vi "Pre Launch Init.vi"(11 "Nested in":refnum<class "Measurement GEN.lvclass">) -> (0 "error out":errorcluster, 3 "Nested out":refnum<class "Measurement GEN.lvclass">)   [LabVIEW 2020, in "Measurement GEN.lvlib" / "Measurement GEN.lvclass"]
doc: "(<B>Filename</B>: Actor Framework.lvlib:Actor.lvclass:Pre Launch Init.vi)\n\nDefines behavior that occurs after the Launch Nested Actor method is invoked but before the actor's Actor Core method begins running.\n\nBy default, this method does nothing. A descendant class may override it to define behavior."
uses:
  Measurement GEN.lvclass
  Measurement GEN.lvclass/Measurement GEN.ctl
  <vilib>/ActorFramework/Actor/Actor.lvclass
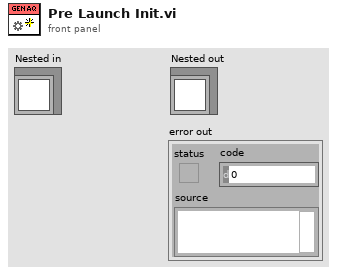
[diagram p1: front panel]
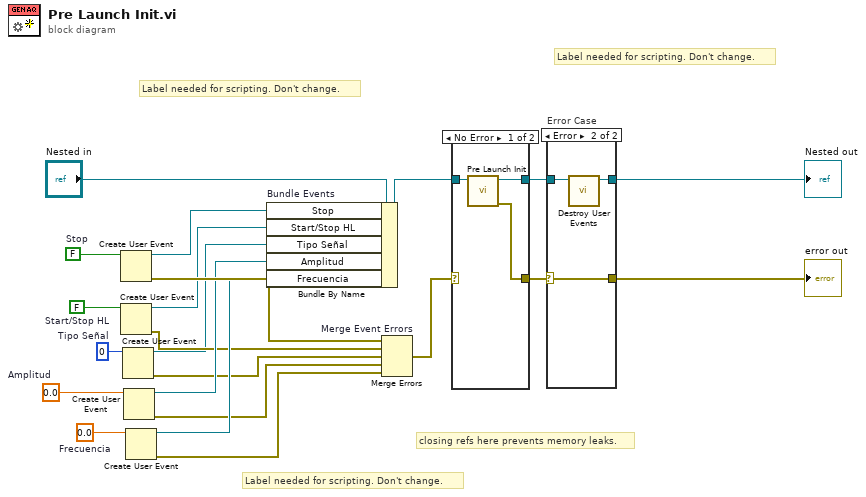
[diagram p0: block diagram]
diagram:
  w2 = u16 0  # Tipo Señal
  w11 = 0.0  # Frecuencia
  w12 = 0.0  # Amplitud
  w13 = FALSE  # Start/Stop HL
  w21 = FALSE  # Stop
  # "Label needed for scripting. Don't change."
  # "Label needed for scripting. Don't change."
  # "Label needed for scripting. Don't change."
  # "closing refs here prevents memory leaks."
  n1 = Create User Event(user event datatype=w21) -> (user event=w10:refnum<user-event>, error out=w20:errorcluster)  [unwired: 1 in]
  n2 = Create User Event(user event datatype=w13) -> (user event=w9:refnum<user-event>, error out=w6:errorcluster)  [unwired: 1 in]
  n3 = Create User Event(user event datatype=w2) -> (user event=w1:refnum<user-event>, error out=w5:errorcluster)  [unwired: 1 in]
  n4 = Create User Event(user event datatype=w12) -> (user event=w8:refnum<user-event>, error out=w4:errorcluster)  [unwired: 1 in]
  n5 = Create User Event(user event datatype=w11) -> (user event=w7:refnum<user-event>, error out=w3:errorcluster)  [unwired: 1 in]
  n6 = Bundle By Name "Bundle Events"(cluster="Nested in", "Stop"=w10, "Start/Stop HL"=w9, "Tipo Señal"=w1, "Amplitud"=w8, "Frecuencia"=w7) -> (w16:refnum<class "Measurement GEN.lvclass">)
  n7 = Merge Errors "Merge Event Errors"(w20, w6, w5, w4, w3) -> (w15:errorcluster)
  n8 = case shown="No Error" w15 {
    selector: w15 -> [_ w27]
    tunnel: [w25 w26] -> w17
    tunnel: w16 -> [w24 w26]
    tunnel: [w23 w27] -> w14
    frame No Error {
      n9 = call-parent "Pre Launch Init.vi"("Actor in"=w24) -> ("error out"=w23:errorcluster, "Actor out"=w25:refnum<class "Measurement GEN.lvclass">)  [unwired: 9 in]
    }
    frame Error {
    }
  }
  n10 = case "Error Case" shown="Error" w14 {
    selector: w14 -> [w28 w32]
    tunnel: w17 -> [w29 w31]
    tunnel: [w29 w30] -> w19
    tunnel: [w28 w32] -> w18
    frame No Error {
    }
    frame Error {
      n11 = call "Destroy User Events.vi"("UI Template in"=w31) -> ("UI Template out"=w30:refnum<class "Measurement GEN.lvclass">)  [unwired: 10 in]
    }
  }
  "error out" <- w18
  "Nested out" <- w19
